vi "Load Start Choice.vi"(11 "Folder Name In":string) -> (1 "Toolkit Name":string, 3 "Target Name":string)   [LabVIEW 2021]
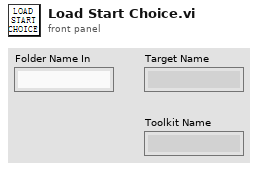
[diagram p1: front panel]
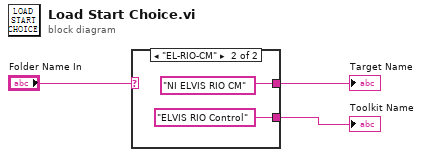
[diagram p0: block diagram]
diagram:
  n1 = case shown="\"EL-RIO-CM\"" "Folder Name In" {
    selector: "Folder Name In" -> [w4 _]
    tunnel: [w4 "NI ELVIS RIO CM"] -> w1
    tunnel: [w4 "ELVIS RIO Control"] -> w3
    frame Default {
    }
    frame "EL-RIO-CM" {
    }
  }
  "Toolkit Name" <- w3
  "Target Name" <- w1
